vi "LEP_RV_GetTargetName.vi"(8 "error in (no error)":errorcluster) -> (0 "error out":errorcluster, 3 "Target Name":string)   [LabVIEW 2011]
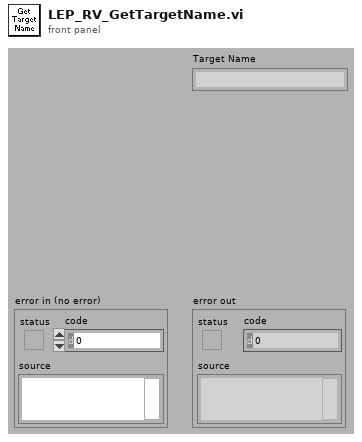
[diagram p1: front panel]
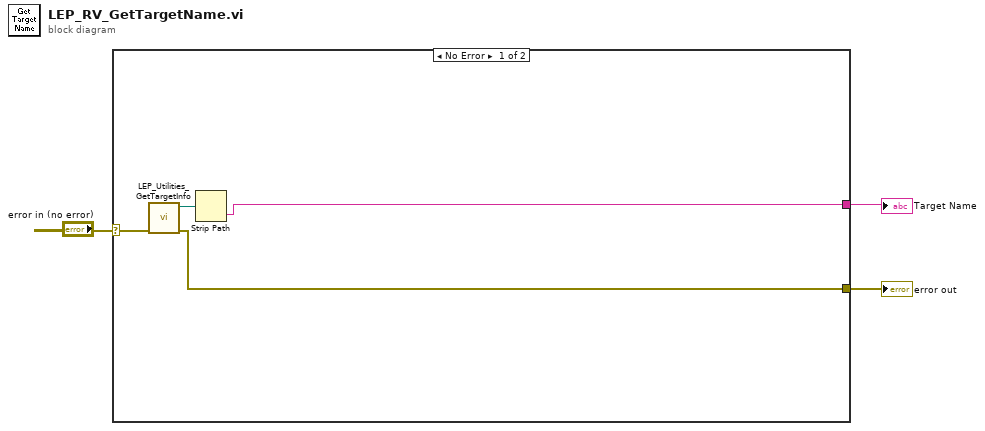
[diagram p0: block diagram]
diagram:
  n1 = case shown="No Error" "error in (no error)" {
    selector: "error in (no error)" -> [w6 w8]
    tunnel: [w5 w8] -> w2
    tunnel: [w4 _] -> w1
    frame No Error {
      n2 = call <vilib>:"LEP_Utilities_GetTargetInfo.vi"("error in"=w6) -> ("error out"=w5:errorcluster, "path"=w7:path)  [unwired: 7 in, 2 out]
      n3 = Strip Path(path=w7) -> (name=w4:string)  [unwired: 1 out]
    }
    frame Error {
    }
  }
  "error out" <- w2
  "Target Name" <- w1
